vi "Log Daemon Message.vi"(8 "error in (no error)":errorcluster, 10 "Line":string, 11 "Engine in":refnum<class "Engine.lvclass">) -> (0 "error out":errorcluster, 3 "Engine out":refnum<class "Engine.lvclass">)   [LabVIEW 2020, in "TSS.lvlib" / "Engine.lvclass"]
uses:
  Engine.lvclass
  Engine.lvclass/Engine.ctl
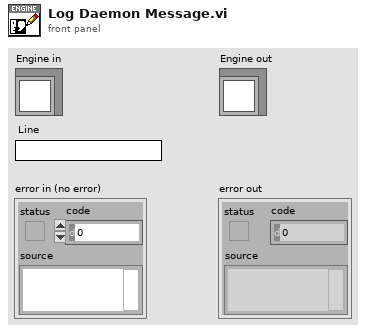
[diagram p1: front panel]
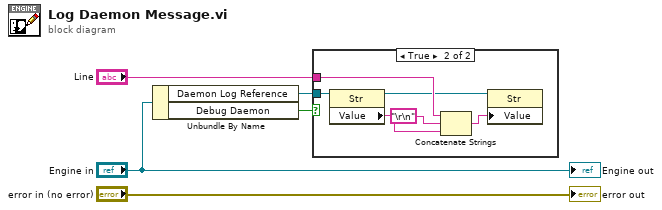
[diagram p0: block diagram]
diagram:
  n1 = Unbundle By Name("Engine in") -> ("Daemon Log Reference"=w3:refnum<vi>, "Debug Daemon"=w1:bool)
  n2 = case shown="True" w1 {
    tunnel: w3 -> [_ w11]
    tunnel: "Line" -> [_ w8]
    frame False {
    }
    frame True {
      n3 = property class="Str"(reference=w11) -> (reference out=w7:refnum<vi>, "Value"=w10:string)  [unwired: 1 in, 1 out]
      n4 = Concatenate Strings(w8, "\r\n", w10) -> (w6:string)
      n5 = property class="Str"(reference=w7, "Value"=w6) -> ()  [unwired: 1 in, 2 out]
    }
  }
  "error out" <- "error in (no error)"
  "Engine out" <- "Engine in"
